vi "MakeExample.vi"(8 "error in (no error)":errorcluster, 9 "TriggerRefractoryPeriod (Frames)":i32, 10 "StimulusObject Parameters":variant, 11 "DetectSuppressionDuration in":refnum<class "DetectSuppressionDuration.lvclass">) -> (0 "error out":errorcluster, 3 "DetectSuppressionDuration out":refnum<class "DetectSuppressionDuration.lvclass">)   [LabVIEW 2019, in "DetectSuppressionDuration.lvclass"]
uses:
  DetectSuppressionDuration.lvclass
  DetectSuppressionDurationInputCluster.ctl
  DetectSuppressionDuration.lvclass/DetectSuppressionDuration.ctl
  ParametersGlobal.vi
  StimulusObject.lvclass
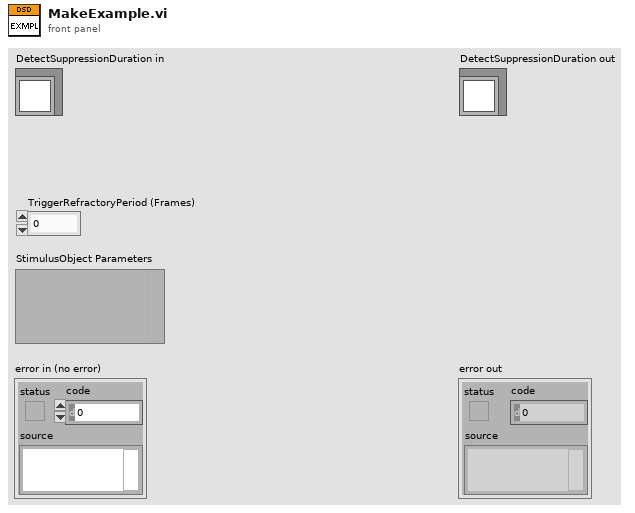
[diagram p1: front panel]
types:
  T1 = typedef "DetectSuppressionDuration.lvclass/DetectSuppressionDurationInputCluster.ctl" = cluster{"Constant Intensity (uW/mm^2, negative is blue)":sgl, "dot radius (mm)":sgl, "Intensities (uW/mm^2, negative is blue)":sgl[], "Durations (s)":sgl[], "Inter trigger interval (s)":dbl, "Ellipse Ratio Trigger Point":sgl, "Delays (s)":sgl[]}
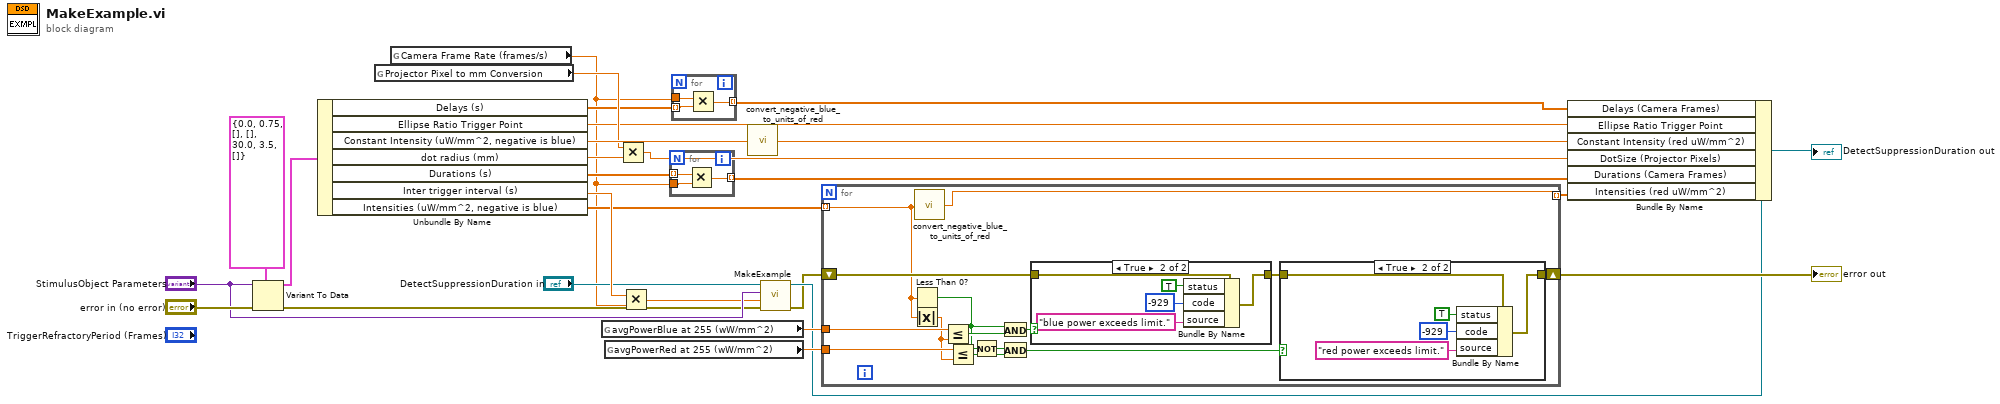
[diagram p0: block diagram]
diagram:
  n1 = Variant To Data(error in="error in (no error)", type=T1 {"Constant Intensity (uW/mm^2, negative is blue)"=0.0, "dot radius (mm)"=0.75, "Intensities (uW/mm^2, negative is blue)"=[], "Durations (s)"=[], "Inter trigger interval (s)"=30.0, "Ellipse Ratio Trigger Point"=3.5, "Delays (s)"=[]} ("DetectSuppressionDurationInputCluster"), Variant="StimulusObject Parameters") -> (data=w27:T1, error out=w5:errorcluster)
  n2 = Unbundle By Name(w27) -> ("Delays (s)"=w3:sgl[], "Ellipse Ratio Trigger Point"=w13:sgl, "Constant Intensity (uW/mm^2, negative is blue)"=w25:sgl, "dot radius (mm)"=w23:sgl, "Durations (s)"=w20:sgl[], "Inter trigger interval (s)"=w26:dbl, "Intensities (uW/mm^2, negative is blue)"=w18:sgl[])
  n3 = global read "ParametersGlobal.vi" "Projector Pixel to mm Conversion"() -> (w22:sgl)
  n4 = global read "ParametersGlobal.vi" "Camera Frame Rate (frames/s)"() -> (w2:sgl)
  n5 = global read "ParametersGlobal.vi" "avgPowerBlue at 255 (wW/mm^2)"() -> (w17:sgl)
  n6 = global read "ParametersGlobal.vi" "avgPowerRed at 255 (wW/mm^2)"() -> (w16:sgl)
  n7 = Multiply(x=w22, y=w23) -> (x*y=w21:sgl)
  n8 = Multiply(x=w26, y=w2) -> (x*y=w6:dbl)
  n9 = for {
    tunnel: w20 -> [w30] mode=indexing
    tunnel: w2 -> [w29]
    tunnel: [w28] -> w19 mode=indexing
    n10 = Multiply(x=w30, y=w29) -> (x*y=w28:sgl)
  }
  n11 = for {
    tunnel: w2 -> [w33]
    tunnel: w3 -> [w32] mode=indexing
    tunnel: [w31] -> w1 mode=indexing
    n12 = Multiply(x=w33, y=w32) -> (x*y=w31:sgl)
  }
  n13 = call "convert_negative_blue_to_units_of_red.vi"("Intensity in units of red (positive) and blue (negative)"=w25) -> ("Intensity in units of red (positive and negative)"=w24:sgl)
  n14 = call-parent "MakeExample.vi"("error in (no error)"=w5, "TriggerRefractoryPeriod (Frames)"=w6, "StimulusObject Parameters"="StimulusObject Parameters", "StimulusObject in"="DetectSuppressionDuration in") -> ("error out"=w4:errorcluster, "StimulusObject out"=w8:refnum<class "DetectSuppressionDuration.lvclass">)  [unwired: 6 in]
  n15 = for {
    tunnel: w18 -> [w41] mode=indexing
    shift-right: [w45] -> w10
    shift-left: w4 -> [w46]
    tunnel: w17 -> [w44]
    tunnel: w16 -> [w43]
    tunnel: [w42] -> w15 mode=indexing
    n16 = Less Than 0?(x=w41) -> (x < 0?=w34:bool)
    n17 = Absolute Value(x=w41) -> (abs(x)=w40:sgl)
    n18 = call "convert_negative_blue_to_units_of_red.vi"("Intensity in units of red (positive) and blue (negative)"=w41) -> ("Intensity in units of red (positive and negative)"=w42:sgl)
    n19 = Less Or Equal?(x=w44, y=w40) -> (x <= y?=w39:bool)
    n20 = Less Or Equal?(x=w43, y=w40) -> (x <= y?=w36:bool)
    n21 = Not(x=w34) -> (.not. x?=w35:bool)
    n22 = And(x=w34, y=w39) -> (x .and. y?=w38:bool)
    n23 = And(x=w35, y=w36) -> (x .and. y?=w37:bool)
    n24 = case shown="True" w38 {
      tunnel: w46 -> [w54 w59]
      tunnel: [w54 w58] -> w47
      frame False {
      }
      frame True {
        n25 = Bundle By Name(cluster=w59, "status"=TRUE, "code"=-929, "source"="blue power exceeds limit.") -> (w58:errorcluster)
      }
    }
    n26 = case shown="True" w37 {
      tunnel: w47 -> [w48 w53]
      tunnel: [w48 w52] -> w45
      frame False {
      }
      frame True {
        n27 = Bundle By Name(cluster=w53, "status"=TRUE, "code"=-929, "source"="red power exceeds limit.") -> (w52:errorcluster)
      }
    }
  }
  "error out" <- w10
  n28 = Bundle By Name(cluster=w8, "Delays (Camera Frames)"=w1, "Ellipse Ratio Trigger Point"=w13, "Constant Intensity (red uW/mm^2)"=w24, "DotSize (Projector Pixels)"=w21, "Durations (Camera Frames)"=w19, "Intensities (red uW/mm^2)"=w15) -> (→"DetectSuppressionDuration out":refnum<class "DetectSuppressionDuration.lvclass">)
